vi "LVObject to JSON - 4D String Array - Returns Error.vi"() -> ()   [LabVIEW 2017, in "Tests.lvlib"]
uses:
  Tests.lvlib
  Flatten To JSON Object/Flatten To JSON Object.lvclass
  4D String Array/4D String Array.lvclass
  <vilib>/addons/_JKI Toolkits/Caraya/classes/Assert/Assert Error.vi
  <vilib>/addons/_JKI Toolkits/Caraya/classes/Test/Test.lvclass
  <vilib>/addons/_JKI Toolkits/Caraya/classes/Assert/Assert.lvclass
panel:
  out "error out":errorcluster
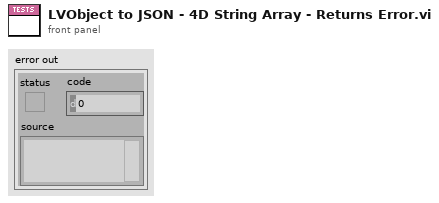
[diagram p1: front panel]
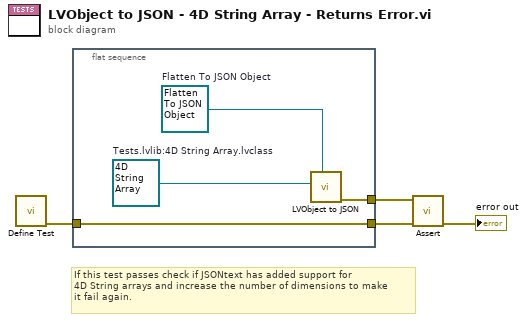
[diagram p0: block diagram]
diagram:
  # "If this test passes check if JSONtext has added support for\n4D String arrays and increase the number of dimensions to make\nit fail again."
  n1 = call <vilib>:"Define Test.vi"() -> ("error out"=w3:errorcluster)  [unwired: 11 in]
  n2 = flat-sequence {
    tunnel: w3 -> [w6]
    tunnel: [w6] -> w2
    tunnel: [w5] -> w1
    frame #0 {
      w7 = refnum<class "4D String Array.lvclass"> refnum  # Tests.lvlib:4D String Array.lvclass
      w8 = refnum<class "Flatten To JSON Object.lvclass"> refnum  # Flatten To JSON Object
      n3 = call-dynamic "LVObject to JSON.vi"("LVClass Serializer"=w8, "Object"=w7) -> ("error out"=w5:errorcluster)  [unwired: 8 in, 1 out]
    }
  }
  n4 = call-poly <vilib>:"Assert.vi"("error in (no error)"=w2, "Error?"=w1) -> ("error out"=→"error out":errorcluster)  [unwired: 9 in]
